vi "create default cache.vi"() -> (3 "cache":T1)   [LabVIEW 2013, in "PL_class cache.lvlib"]
uses:
  PL_class cache.lvlib
  cache definition.ctl
  class metadata.ctl
  class type.ctl
  <vilib>/Utility/libraryn.llb/Check if File or Folder Exists.vi
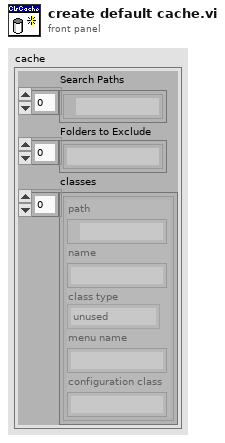
[diagram p1: front panel]
types:
  T1 = typedef "PL_class cache.lvlib/cache definition.ctl" = cluster{"Search Paths":path[], "Folders to Exclude":string[], "classes":T2[]}
  T2 = typedef "PL_class cache.lvlib/class metadata.ctl" = cluster{"path":path, "name":string, "class type":T3, "menu name":string, "configuration class":string}
  T3 = typedef "PL_class cache.lvlib/class type.ctl" = enum16{"unused", "other pl", "system", "target", "engine", "module"}
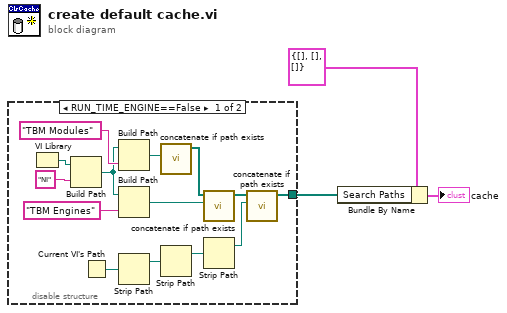
[diagram p0: block diagram]
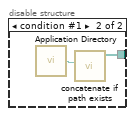
[diagram p2: hidden frame]
diagram:
  n1 = disable-structure shown="RUN_TIME_ENGINE==False" {
    disable-tunnel: [w8 w18] -> w3
    frame condition #0 (active) {
      n2 = VI Library() -> (path=w17:path)
      n3 = Build Path(base path=w17, name or relative path="NI") -> (appended path=w13:path)
      n4 = Current VI's Path() -> (path=w7:path)
      n5 = Build Path(base path=w13, name or relative path="TBM Modules") -> (appended path=w10:path)
      n6 = Build Path(base path=w13, name or relative path="TBM Engines") -> (appended path=w11:path)
      n7 = Strip Path(path=w7) -> (stripped path=w6:path)  [unwired: 1 out]
      n8 = call "concatenate if path exists.vi"("new path"=w10) -> ("paths out"=w12:path[])  [unwired: 10 in]
      n9 = Strip Path(path=w6) -> (stripped path=w5:path)  [unwired: 1 out]
      n10 = call "concatenate if path exists.vi"("new path"=w11, "paths in"=w12) -> ("paths out"=w9:path[])  [unwired: 9 in]
      n11 = Strip Path(path=w5) -> (stripped path=w4:path)  [unwired: 1 out]
      n12 = call "concatenate if path exists.vi"("new path"=w4, "paths in"=w9) -> ("paths out"=w8:path[])  [unwired: 9 in]
    }
    frame condition #1 {
      n13 = call <vilib>:"Application Directory.vi"() -> ("Application Directory"=w19:path)
      n14 = call "concatenate if path exists.vi"("new path"=w19) -> ("paths out"=w18:path[])  [unwired: 10 in]
    }
  }
  n15 = Bundle By Name(cluster=T1 {"Search Paths"=[], "Folders to Exclude"=[], "classes"=[]} ("cache"), "Search Paths"=w3) -> (→"cache":T1)
